vi "DataRead1.vi"() -> ()   [LabVIEW 2024]
panel:
  out "Waveform Graph":waveform(dbl)[](graph)
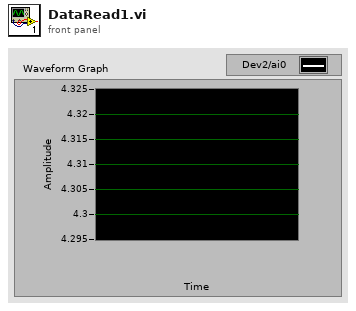
[diagram p1: front panel]
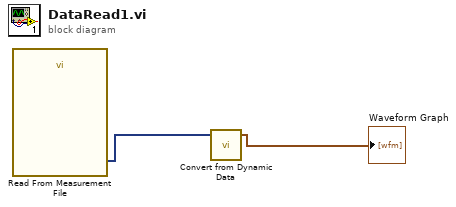
[diagram p0: block diagram]
diagram:
  n1 = call "Read From Measurement File"() -> ("Signals"=w2:dynamicdata)  [unwired: 6 in, 5 out]
  n2 = call "Convert from Dynamic Data"("Dynamic Data Type"=w2) -> ("Array of Waveform"=→"Waveform Graph":waveform(dbl)[])  [unwired: 3 in]
